vi "Get Ring Ctrl Refnum.vi"(8 "error in (no error)":errorcluster, 11 "FK Ring in":refnum<class "FK Ring.lvclass">) -> (0 "error out":errorcluster, 2 "Ring Refnum":refnum<vi>, 3 "FK Ring out":refnum<class "FK Ring.lvclass">)   [LabVIEW 2020, in "Basic Fields.lvlib" / "FK Ring.lvclass"]
uses:
  FK Ring.lvclass
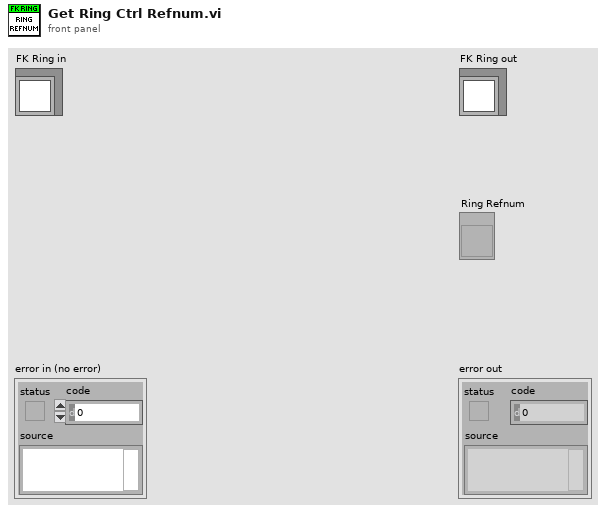
[diagram p1: front panel]
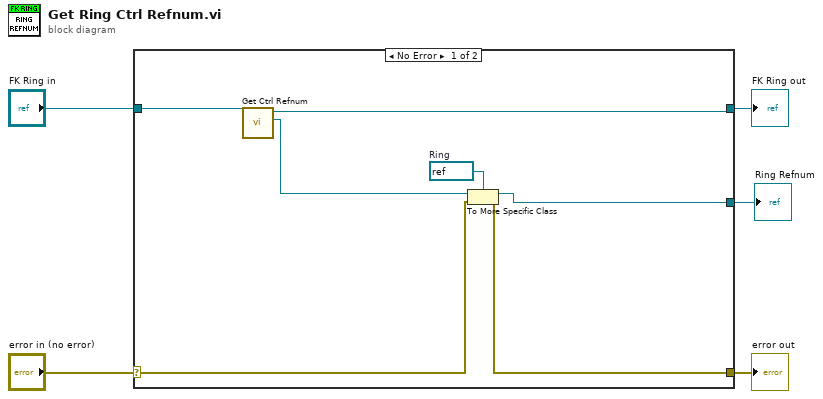
[diagram p0: block diagram]
diagram:
  n1 = case shown="No Error" "error in (no error)" {
    selector: "error in (no error)" -> [w6 w14]
    tunnel: [w10 w14] -> w4
    tunnel: [w7 w13] -> w2
    tunnel: "FK Ring in" -> [w9 w13]
    tunnel: [w11 _] -> w1
    frame No Error {
      w12 = refnum<vi> refnum  # Ring
      n2 = call-dynamic "Get Ctrl Refnum.vi"("Ctrl Refnum Column in"=w9) -> ("Ctl Refnum"=w8:refnum<vi>, "Ctrl Refnum Column out"=w7:refnum<class "FK Ring.lvclass">)  [unwired: 8 in, 1 out]
      n3 = To More Specific Class(target class=w12, reference=w8, error in=w6) -> (specific class reference=w11:refnum<vi>, error out=w10:errorcluster)
    }
    frame Error {
    }
  }
  "error out" <- w4
  "FK Ring out" <- w2
  "Ring Refnum" <- w1
